vi "line-follower.vi"   [LabVIEW 2016, in "LineFollower2Sensor.lvrbt"]
uses:
  LineFollower2Sensor.lvrbt
  <vilib>/NXT/Subs/LVHSConnector.ctl
  <vilib>/NXT/LegoClasses/BrickReference/BrickReference.lvclass
  <vilib>/NXT/Block Support/NXT_ButtonSelector.ctl
  <vilib>/NXT/Block Support/NXT_InputPort.ctl
  <vilib>/NXT/Subs/MotorOutput.ctl
  <vilib>/NXT/Dual Mode Library/Sensors/Color_Detector.vi
  <vilib>/NXT/Dual Mode Library/Waits/Wait_Num.vi
  <vilib>/NXT/Dual Mode Library/Motors/MotorOn.vi
types:
  T1 = typedef "NXT_InputPort.ctl" = u32
  T2 = typedef "LVHSConnector.ctl" = refnum<class "BrickReference.lvclass">
  T3 = typedef "ColorSensorColors.ctl" = enum16{"No Color", "Black", "Blue", "Green", "Yellow", "Red", "White", "Brown"}
  T4 = typedef "MotorOutput.ctl" = u8
  T5 = typedef "NXT_ButtonSelector.ctl" = u16
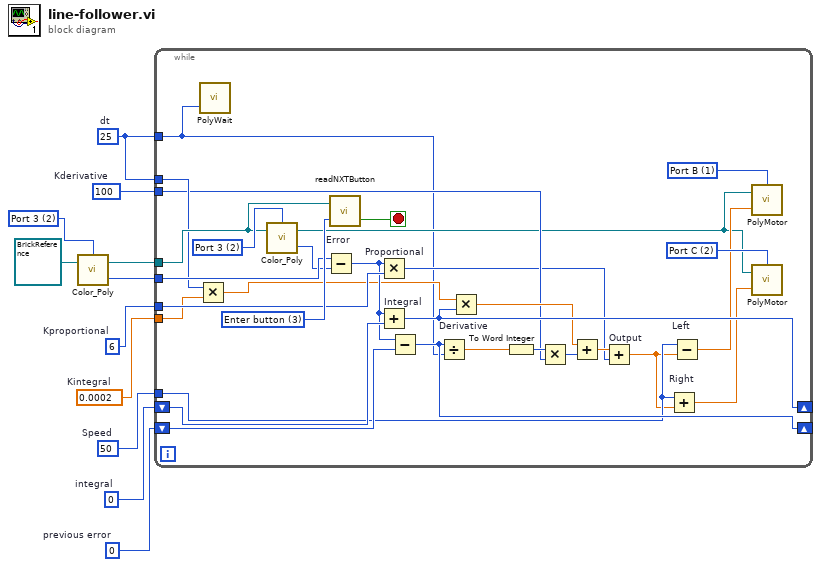
[diagram p0: block diagram]
diagram:
  w1 = i16 50  # Speed
  w5 = i16 0  # integral
  w6 = i16 0  # previous error
  w8 = T1 2 items=["Port 1", "Port 2", "Port 3", "Port 4"] ("Port (Port 3)")
  w3 = i16 25  # dt
  w2 = i16 100  # Kderivative
  w4 = 0.0002  # Kintegral
  w7 = i16 6  # Kproportional
  n1 = call-poly <vilib>:"Color_Poly.vi"("NXT/EV3"=T2 refnum ("NXT"), "Port (Port 3)"=w8) -> ("Detected Color"=w9:T3, "NXT/EV3"=w10:T2)  [unwired: 1 in]
  n2 = while {
    tunnel: w10 -> [w37]
    tunnel: w9 -> [w39]
    tunnel: w7 -> [w35]
    shift-right: [w30] -> _
    shift-left: w6 -> [w32]
    shift-right: [w26] -> _
    shift-left: w5 -> [w34]
    tunnel: w3 -> [w12]
    tunnel: w4 -> [w29]
    tunnel: w3 -> [w28]
    tunnel: w2 -> [w22]
    tunnel: w1 -> [w19]
    stop <- w41 stop-if-true
    w15 = T4 1 items=["Port A"=0, "Port B"=1, "Port C"=2, "Ports A & B"=4, "Ports A & C"=5, "Ports B & C"=6, "All Ports"=3] ("Output Port (All Ports)")
    w17 = T4 2 items=["Port A"=0, "Port B"=1, "Port C"=2, "Ports A & B"=4, "Ports A & C"=5, "Ports B & C"=6, "All Ports"=3] ("Output Port (All Ports)")
    w38 = T1 2 items=["Port 1", "Port 2", "Port 3", "Port 4"] ("Port (Port 3)")
    w40 = T5 3 items=["Enter button"=3, "Left button"=2, "Right button"=1] ("Button (Enter button)")
    n3 = Multiply(x=w28, y=w29) -> (x*y=w27:dbl)
    n4 = call-poly <vilib>:"PolyWait.vi"("Time (1 sec)"=w12) -> ()  [unwired: 3 in, 1 out]
    n5 = call-poly <vilib>:"Color_Poly.vi"("NXT/EV3"=w37, "Port (Port 3)"=w38) -> ("Detected Color"=w36:T3, "NXT/EV3"=w13:T2)  [unwired: 1 in]
    n6 = Subtract "Error"(x=w39, y=w36) -> (x-y=w33:u16)
    n7 = call <vilib>:"readNXTButton.vi"("Button (Enter button)"=w40, "NXT/EV3"=w37) -> ("Yes/No"=w41:bool)  [unwired: 1 in, 1 out]
    n8 = Multiply "Proportional"(x=w33, y=w35) -> (x*y=w20:u16)
    n9 = Add "Integral"(x=w33, y=w34) -> (x+y=w26:u16)
    n10 = Subtract(x=w33, y=w32) -> (x-y=w30:u16)
    n11 = Divide "Derivative"(x=w30, y=w12) -> (x/y=w31:dbl)
    n12 = Multiply(x=w27, y=w26) -> (x*y=w25:dbl)
    n13 = To Word Integer(number=w31) -> (16bit integer=w23:i16)
    n14 = Multiply(x=w23, y=w22) -> (x*y=w24:i16)
    n15 = Add(x=w25, y=w24) -> (x+y=w21:dbl)
    n16 = Add "Output"(x=w21, y=w20) -> (x+y=w18:dbl)
    n17 = Add "Right"(x=w19, y=w18) -> (x+y=w16:dbl)
    n18 = Subtract "Left"(x=w19, y=w18) -> (x-y=w14:dbl)
    n19 = call-poly <vilib>:"PolyMotor.vi"("Power (75)"=w14, "NXT/EV3"=w13, "Output Port (All Ports)"=w15) -> ()  [unwired: 1 in, 1 out]
    n20 = call-poly <vilib>:"PolyMotor.vi"("Power (75)"=w16, "NXT/EV3"=w13, "Output Port (All Ports)"=w17) -> ()  [unwired: 1 in, 1 out]
  }
